vi "observacao_0MQ.vi"() -> ()   [LabVIEW 2012, in "Shared_160.lvlib"] (continued)
                        n2726 = call "Monta Comando.vi"("Set Point"=" 48 00", "Comando"="ESCREVER", "Dispositivo"="TAMPAS" ("Comando"), "Controlador"=w3460) -> ("Resposta"=w3454:string)  [unwired: 3 in, 2 out]
                        n2727 = Tick Count (ms)() -> (millisecond timer value=→"TF2":u32)
                        n2728 = Not Equal?(x=w3454, y="TAMPAS OK") -> ()  [unwired: 1 out]
                        n2729 = Select(t="REPOUSO" ("y"), s=FALSE, f="ESPERA2") -> (s? t:f=w3455:string)
                      }
                      frame "ESPERA2" {
                        # "10 SEGUNDOS"
                        n2730 = local read "TF2"() -> (w3461:u32)
                        n2731 = Tick Count (ms)() -> (millisecond timer value=w3467:u32)
                        n2732 = Add(x=w3461, y=u32 10000) -> (x+y=w3468:u32)
                        n2733 = Greater?(x=w3467, y=w3468) -> (0:w3462:bool)
                        n2734 = Select(t="PIZZA3" ("y"), s=w3462, f="ESPERA2" ("y")) -> (s? t:f=w3463:string)
                      }
                      frame "PIZZA3" {
                        w3479 = u16 3 items=["ZERO", "AH", "DEC", "TUBO", "CUP"] ("Controlador")
                        n2735 = call "Monta Comando.vi"("Set Point"=" 48 48", "Comando"="ESCREVER", "Dispositivo"="TAMPAS" ("Comando"), "Controlador"=w3479) -> ("Resposta"=w3474:string)  [unwired: 3 in, 2 out]
                        n2736 = case shown="True" "Case Constant\n(See Context Help) 12" {
                          frame False {
                          }
                          frame True {
                            n2737 = local write "LED ACTION"(FALSE ("LED ACTION")) -> ()
                          }
                        }
                        n2738 = Not Equal?(x=w3474, y="TAMPAS OK") -> ()  [unwired: 1 out]
                        n2739 = Select(t="REPOUSO" ("y"), s=FALSE, f="REPOUSO" ("y")) -> (s? t:f=w3471:string)
                      }
                      frame "REPOUSO" {
                      }
                    }
                    n2740 = local write "ESTADO FECHAR"(w3370) -> ()
                    n2741 = local read "ESTADO ABRIR"() -> (w3369:string)
                    n2742 = case shown="\"ESPERA3\"" w3369 {
                      tunnel: [w3376 w3384 w3392 w3402 w3411 w3424 "REPOUSO" ("y")] -> w3368
                      frame "INICIO", Default {
                        w3382 = u16 3 items=["ZERO", "AH", "DEC", "TUBO", "CUP"] ("Controlador")
                        # "PASSA PARA MODO HANDSET"
                        n2743 = call "Monta Comando.vi"("Set Point"=" F8 00", "Comando"="ESCREVER", "Dispositivo"="TAMPAS" ("Comando"), "Controlador"=w3382) -> ("Resposta"=w3377:string)  [unwired: 3 in, 2 out]
                        n2744 = Not Equal?(x=w3377, y="TAMPAS OK") -> ()  [unwired: 1 out]
                        n2745 = Tick Count (ms)() -> (millisecond timer value=→"TA1":u32)
                        n2746 = Select(t="REPOUSO" ("y"), s=FALSE, f="ESPERA1" ("y")) -> (s? t:f=w3376:string)
                      }
                      frame "ESPERA1" {
                        # "1 SEGUNDO"
                        n2747 = local read "TA1"() -> (w3383:u32)
                        n2748 = Tick Count (ms)() -> (millisecond timer value=w3389:u32)
                        n2749 = Add(x=w3383, y=u32 1000) -> (x+y=w3388:u32)
                        n2750 = Greater?(x=w3389, y=w3388) -> (0:w3386:bool)
                        n2751 = Select(t="ABREPIZZA" ("y"), s=w3386, f="ESPERA1" ("y")) -> (s? t:f=w3384:string)
                      }
                      frame "ABREPIZZA" {
                        w3401 = u16 3 items=["ZERO", "AH", "DEC", "TUBO", "CUP"] ("Controlador")
                        # "MANDA PIZZA ABRIR"
                        n2752 = call "Monta Comando.vi"("Set Point"=" 48 48", "Comando"="ESCREVER", "Dispositivo"="TAMPAS" ("Comando"), "Controlador"=w3401) -> ("Resposta"=w3396:string)  [unwired: 3 in, 2 out]
                        n2753 = Not Equal?(x=w3396, y="TAMPAS OK") -> ()  [unwired: 1 out]
                        n2754 = Tick Count (ms)() -> (millisecond timer value=→"TA2":u32)
                        n2755 = Select(t="ABREPIZZA" ("y"), s=FALSE, f="ESPERA2" ("y")) -> (s? t:f=w3392:string)
                      }
                      frame "ESPERA2" {
                        # "10 SEGUNDOS"
                        n2756 = local read "TA2"() -> (w3403:u32)
                        n2757 = Tick Count (ms)() -> (millisecond timer value=w3408:u32)
                        n2758 = Add(x=w3403, y=u32 10000) -> (x+y=w3407:u32)
                        n2759 = Greater?(x=w3408, y=w3407) -> (0:w3405:bool)
                        n2760 = Select(t="BACIAABRINDO" ("y"), s=w3405, f="ESPERA2" ("y")) -> (s? t:f=w3402:string)
                      }
                      frame "BACIAABRINDO" {
                        w3420 = u16 3 items=["ZERO", "AH", "DEC", "TUBO", "CUP"] ("Controlador")
                        # "BACIA ABRINDO"
                        n2761 = call "Monta Comando.vi"("Set Point"=" A0 20", "Comando"="ESCREVER", "Dispositivo"="TAMPAS" ("Comando"), "Controlador"=w3420) -> ("Resposta"=w3415:string)  [unwired: 3 in, 2 out]
                        n2762 = Not Equal?(x=w3415, y="TAMPAS OK") -> ()  [unwired: 1 out]
                        n2763 = Tick Count (ms)() -> (millisecond timer value=→"TA3":u32)
                        n2764 = Select(t="BACIAABRINDO" ("y"), s=FALSE, f="ESPERA3" ("y")) -> (s? t:f=w3411:string)
                      }
                      frame "ESPERA3" {
                        # "25 SEGUNDOS"
                        n2765 = local read "TA3"() -> (w3422:u32)
                        n2766 = Tick Count (ms)() -> (millisecond timer value=w3427:u32)
                        n2767 = Add(x=w3422, y=u32 25000) -> (x+y=w3426:u32)
                        n2768 = Greater?(x=w3427, y=w3426) -> (0:w3421:bool)
                        n2769 = case shown="True" w3421 {
                          frame False {
                          }
                          frame True {
                            n2770 = local write "LED ACTION"(TRUE ("LED ACTION")) -> ()
                          }
                        }
                        n2771 = Select(t="REPOUSO" ("y"), s=w3421, f="ESPERA3" ("y")) -> (s? t:f=w3424:string)
                      }
                      frame "REPOUSO" {
                      }
                    }
                    n2772 = local write "ESTADO ABRIR"(w3368) -> ()
                  }
                }
              }
              frame #2 {
                # "MÁQUINA DE ESTADOS PROTEÇÃO"
                n2773 = case shown="3" "M_PROT" {
                  selector: "M_PROT" -> [w3485 _ _ _ _ _]
                  tunnel: [w3485 w3486 w3505 5 5 ("estadoCUP") 0 ("estadoCUP")] -> w3483
                  frame 0, Default {
                    # "Sem movimento"
                    n2774 = call "TickTimeout.vi"() -> ("msTick"=→"Timeout PROT":u32)  [unwired: 2 in, 2 out]
                  }
                  frame 1 {
                    w3489 = u16 3 items=["Alarme", "Atencao", "Erro", "Ocupado", "Protecao", "Embreagem", "Tracking", "Var. Track", "Rápido", "Ligeiro", "Médio", "Lento", "Em movimento", ""] ("NomeStatus")
                    w3488 = u16 3 items=["Alarme", "Atencao", "Erro", "Ocupado", "Protecao", "Embreagem", "Tracking", "Var. Track", "Rápido", "Ligeiro", "Médio", "Lento", "Em movimento", ""] ("NomeStatus")
                    # "Testa Ocupado"
                    n2775 = call "Bit Status DEC.vi"("NomeStatus"=w3488) -> ("StatBit"=w3490:bool)
                    n2776 = call "Bit Status AH.vi"("NomeStatus"=w3489) -> ("StatBit"=w3491:bool)
                    n2777 = Or(x=w3491, y=w3490) -> (x .or. y?=w3487:bool)
                    n2778 = case shown="False" w3487 {
                      tunnel: [2 w3502] -> w3486
                      frame False {
                        w3498 = u16 2 items=["ZERO", "AH", "DEC", "TUBO", "CUP"] ("Controlador")
                        w3493 = u16 1 items=["ZERO", "AH", "DEC", "TUBO", "CUP"] ("Controlador")
                        # "Comando para os controladores\nsaírem da Proteção"
                        n2779 = call "Monta Comando.vi"("Comando"="LIBERAR", "Dispositivo"="EIXO" ("Comando"), "Controlador"=w3493) -> ()  [unwired: 4 in, 3 out]
                        n2780 = call "Monta Comando.vi"("Comando"="LIBERAR", "Dispositivo"="EIXO" ("Comando"), "Controlador"=w3498) -> ()  [unwired: 4 in, 3 out]
                      }
                      frame True {
                        # "Busy"
                        n2781 = local read "Timeout PROT"() -> (w3501:u32)
                        n2782 = call "TickTimeout.vi"("msInicial"=w3501, "msTimeout"=u32 20000) -> ("Timeout"=w3499:bool)  [unwired: 2 out]
                        n2783 = case shown="False" w3499 {
                          tunnel: [1 3] -> w3502
                          frame False {
                          }
                          frame True {
                          }
                        }
                      }
                    }
                  }
                  frame 2 {
                    # "Cálculos rápidos"
                    # "Vem do Setup"
                    # "Aguarda Sair da proteção"
                    n2784 = global read "Global_Telescopio.vi" "Zenital angle GRAUS"() -> (w3508:dbl)
                    n2785 = global read "Global_Telescopio.vi" "Z_LIBERA_GRAUS"() -> (w3507:dbl)
                    n2786 = Less?(x=w3508, y=w3507) -> (x < y?=w3506:bool)
                    n2787 = case shown="True" w3506 {
                      tunnel: [2 ("estadoCUP") 4 ("estadoCUP")] -> w3505
                      frame False {
                      }
                      frame True {
                        # "stop"
                      }
                    }
                  }
                  frame 3 {
                    w3511 = "TENTE NOVAMENTE" ("SYSTEM MESSAGES")
                    # "Trata Timeout"
                    n2788 = call "TickTimeout.vi"() -> ("msTick"=w3512:u32)  [unwired: 2 in, 2 out]
                    n2789 = call "Monta_Mensagem.vi"("Mensagem"=w3511) -> ()  [unwired: 2 in]
                    n2790 = call "Salva_systems_messages.vi"("Mensagem"=w3511) -> ()  [unwired: 5 in]
                    n2791 = local write "Timeout PROT"(w3512) -> ()
                  }
                  frame 4 {
                    w3515 = u16 1 items=["ZERO", "AH", "DEC", "TUBO", "CUP"] ("Controlador")
                    w3520 = u16 2 items=["ZERO", "AH", "DEC", "TUBO", "CUP"] ("Controlador")
                    # "Para os motores"
                    n2792 = call "Monta Comando.vi"("Comando"="PARAR", "Dispositivo"="PROG", "Controlador"=w3515) -> ()  [unwired: 4 in, 3 out]
                    n2793 = call "Monta Comando.vi"("Comando"="PARAR", "Dispositivo"="PROG", "Controlador"=w3520) -> ()  [unwired: 4 in, 3 out]
                  }
                  frame 5 {
                    # "SAÍDA"
                  }
                }
                n2794 = local write "M_PROT"(w3483) -> ()
              }
              frame #3 {
                w3539 = u16 3 items=["Alarme", "Atencao", "Erro", "Ocupado", "TBD", "LCB", "Trapeira", "Paravento", "DomoRap", "DomoCW", "DomoCCW", "TBD", "Em movimento", "TBD"] ("NomeStatus")
                w3545 = u16 3 items=["Alarme", "Atencao", "Erro", "Ocupado", "Protecao", "Embreagem", "Tracking", "Var. Track", "Rápido", "Ligeiro", "Médio", "Lento", "Em movimento", ""] ("NomeStatus")
                w3546 = u16 3 items=["Alarme", "Atencao", "Erro", "Ocupado", "Protecao", "Embreagem", "Tracking", "Var. Track", "Rápido", "Ligeiro", "Médio", "Lento", "Em movimento", ""] ("NomeStatus")
                n2795 = global read "Global_Telescopio.vi" "LimiarRapMed"() -> (w3547:dbl)
                n2796 = global read "Global_Telescopio.vi" "PosAH"() -> (w3549:dbl)
                n2797 = global read "Global_Telescopio.vi" "ErroMaxEixo"() -> (w3544:dbl)
                n2798 = global read "Global_Telescopio.vi" "PosDEC"() -> (w3548:dbl)
                n2799 = call "Bit Status DEC.vi"("NomeStatus"=w3545) -> ("StatBit"=w3543:bool)
                n2800 = call "Bit Status AH.vi"("NomeStatus"=w3546) -> ("StatBit"=w3542:bool)
                n2801 = case shown="4" "M_DEC" {
                  selector: "M_DEC" -> [w3642 _ _ _ _ _ _ _ _]
                  tunnel: [w3642 w3648 w3675 w3700 w3723 w3747 0 w3764 w3769] -> w3528
                  tunnel: "DestDEC" -> [_ w3647 w3672 w3694 w3720 _ _ _ _]
                  tunnel: w3548 -> [_ w3650 _ w3697 _ _ _ _ _]
                  tunnel: w3544 -> [_ _ _ w3698 _ _ _ _ _]
                  tunnel: w3547 -> [_ w3649 _ _ _ _ _ _ _]
                  tunnel: w3543 -> [_ w3646 _ w3693 _ _ _ _ _]
                  frame 0, Default {
                    w3640 = 0 ("CR DEC")
                    # "Sem apontamento"
                    n2802 = call "TickTimeout.vi"() -> ("msTick"=→"TimeoutDEC 2":u32)  [unwired: 2 in, 2 out]
                    "CR DEC UTILS" <- w3640
                    "CONT DEC UTILS" <- w3640
                  }
                  frame 1 {
                    # "Envia\nComando"
                    n2803 = Subtract(x=w3647, y=w3650) -> (x-y=w3645:dbl)
                    n2804 = Absolute Value(x=w3645) -> (abs(x)=w3651:dbl)
                    n2805 = Less?(x=w3651, y=w3649) -> (x < y?=w3644:bool)
                    n2806 = case shown="False" w3644 {
                      tunnel: [w3655 3] -> w3648
                      tunnel: w3647 -> [w3654 _]
                      tunnel: w3645 -> [w3653 _]
                      tunnel: w3646 -> [w3652 _]
                      frame False {
                        # "destino"
                        # "Fora do"
                        n2807 = case shown="False" w3652 {
                          tunnel: [20 w3664] -> w3655
                          tunnel: w3654 -> [w3658 _]
                          tunnel: w3653 -> [_ _]
                          frame False {
                            w3662 = u16 2 items=["ZERO", "AH", "DEC", "TUBO", "CUP"] ("Controlador")
                            # "CLP Pronto"
                            n2808 = local write "DEC on Target"(FALSE ("DEC on Target")) -> ()
                            n2809 = call "rad_hms.vi"("TRUE=HORA\nFALSE=GRAU"=FALSE, "Radiano"=w3658) -> ("Hora/Graus Texto Decimal"=w3659:string)  [unwired: 3 in]
                            n2810 = call "Monta Comando.vi"("Set Point"=w3659, "Comando"="MOVER_RAP", "Dispositivo"="EIXO" ("Comando"), "Controlador"=w3662) -> ()  [unwired: 3 in, 3 out]
                          }
                          frame True {
                            # "CLP Ocupado"
                            n2811 = local read "TimeoutDEC 2"() -> (w3666:u32)
                            n2812 = call "TickTimeout.vi"("msInicial"=w3666, "msTimeout"=u32 4000) -> ("Timeout"=w3665:bool)  [unwired: 2 out]
                            n2813 = case shown="False" w3665 {
                              tunnel: [1 5] -> w3664
                              frame False {
                              }
                              frame True {
                                # "Tratar\nTimeout"
                              }
                            }
                          }
                        }
                      }
                      frame True {
                        # "Dist. pequena p/ mov. rápido"
                        # "Ligar mov. lento"
                        n2814 = call "TickTimeout.vi"() -> ("msTick"=w3670:u32)  [unwired: 2 in, 2 out]
                        n2815 = local write "TimeoutDEC 2"(w3670) -> ()
                      }
                    }
                    n2816 = local write "dec="(FALSE ("dec=")) -> ()
                  }
                  frame 2 {
                    w3678 = u16 12 items=["Alarme", "Atencao", "Erro", "Ocupado", "Protecao", "Embreagem", "Tracking", "Var. Track", "Rápido", "Ligeiro", "Médio", "Lento", "Em movimento", ""] ("NomeStatus")
                    # "Aguarda fim mov. Rap."
                    n2817 = call "Bit Status DEC.vi"("NomeStatus"=w3678) -> ("StatBit"=w3679:bool)
                    n2818 = case shown="False" w3679 {
                      tunnel: [1 w3688] -> w3676
                      tunnel: w3672 -> [_ w3687]
                      frame False {
                        # "Motor parado.\nTestar se chegou\nao destino"
                        n2819 = call "TickTimeout.vi"() -> ("msTick"=w3684:u32)  [unwired: 2 in, 2 out]
                        n2820 = local write "TimeoutDEC 2"(w3684) -> ()
                      }
                      frame True {
                        # "Ainda movendo...\nAGUARDAR"
                        n2821 = call "PROTECAO_DEC_UTILS.vi"("Destino DEC"=w3687) -> ("CONT DEC"=w3686:i32)  [unwired: 10 in]
                        n2822 = local read "Erro PROTEC"() -> (w3689:i32)
                        n2823 = Greater Or Equal?(x=w3686, y=w3689) -> (x >= y?=w3692:bool)
                        n2824 = local write "CONT DEC UTILS"(w3686) -> ()
                        n2825 = Select(t=6, s=w3692, f=2) -> (s? t:f=w3688:i32)
                      }
                    }
                    n2826 = global read "Global_Telescopio.vi" "Habilita supervisao"() -> (w3674:bool)
                    n2827 = case shown="True" w3674 {
                      tunnel: [FALSE w3683] -> w3673
                      frame False {
                      }
                      frame True {
                        n2828 = local read "CR DEC UTILS"() -> (w3681:i32)
                        n2829 = local read "Erro Lim"() -> (w3682:i32)
                        n2830 = Greater Or Equal?(x=w3681, y=w3682) -> (x >= y?=w3683:bool)
                      }
                    }
                    n2831 = Select(t=6, s=w3673, f=w3676) -> (s? t:f=w3675:i32)
                  }
                  frame 3 {
                    # "Mov.Lento"
                    n2832 = Subtract(x=w3694, y=w3697) -> (x-y=w3695:dbl)
                    n2833 = Absolute Value(x=w3695) -> (abs(x)=w3699:dbl)
                    n2834 = Less Or Equal?(x=w3699, y=w3698) -> (x <= y?=w3696:bool)
                    n2835 = case shown="False" w3696 {
                      tunnel: [w3702 0] -> w3700
                      tunnel: w3695 -> [w3701 _]
                      tunnel: w3693 -> [w3703 _]
                      frame False {
                        n2836 = case shown="False" w3703 {
                          tunnel: [40 w3712] -> w3702
                          tunnel: w3701 -> [w3706 _]
                          frame False {
                            w3711 = u16 2 items=["ZERO", "AH", "DEC", "TUBO", "CUP"] ("Controlador")
                            # "Mov. lento"
                            n2837 = call "TickTimeout.vi"() -> ("msTick"=w3704:u32)  [unwired: 2 in, 2 out]
                            n2838 = local write "TimeoutDEC 2"(w3704) -> ()
                            n2839 = call "rad_hms.vi"("TRUE=HORA\nFALSE=GRAU"=FALSE ("TRUE=HORA\nFALSE=GRAU"), "Radiano"=w3706) -> ("Hora/Graus Texto Decimal"=w3708:string)  [unwired: 3 in]
                            n2840 = call "Monta Comando.vi"("Set Point"=w3708, "Comando"="MOVER_REL", "Dispositivo"="EIXO" ("Comando"), "Controlador"=w3711) -> ()  [unwired: 3 in, 3 out]
                          }
                          frame True {
                            # "CLP Ocupado"
                            n2841 = local read "TimeoutDEC 2"() -> (w3714:u32)
                            n2842 = call "TickTimeout.vi"("msInicial"=w3714, "msTimeout"=u32 2000) -> ("Timeout"=w3713:bool)  [unwired: 2 out]
                            n2843 = case shown="False" w3713 {
                              tunnel: [3 5] -> w3712
                              frame False {
                              }
                              frame True {
                              }
                            }
                          }
                        }
                      }
                      frame True {
                        # "DEC no destino"
                        n2844 = local write "DEC on Target"(TRUE ("DEC on Target")) -> ()
                      }
                    }
                  }
                  frame 4 {
                    w3726 = u16 12 items=["Alarme", "Atencao", "Erro", "Ocupado", "Protecao", "Embreagem", "Tracking", "Var. Track", "Rápido", "Ligeiro", "Médio", "Lento", "Em movimento", ""] ("NomeStatus")
                    # "Aguarda fim mov. lento"
                    n2845 = global read "Global_Telescopio.vi" "Habilita supervisao"() -> (w3725:bool)
                    n2846 = call "Bit Status DEC.vi"("NomeStatus"=w3726) -> ("StatBit"=w3727:bool)
                    n2847 = case shown="True" w3727 {
                      tunnel: [3 w3737] -> w3722
                      tunnel: w3720 -> [_ w3735]
                      frame False {
                        # "Motor parado.\nTestar se chegou\nao destino"
                        n2848 = call "TickTimeout.vi"() -> ("msTick"=w3732:u32)  [unwired: 2 in, 2 out]
                        n2849 = local write "TimeoutDEC 2"(w3732) -> ()
                      }
                      frame True {
                        n2850 = call "PROTECAO_DEC_UTILS.vi"("Destino DEC"=w3735) -> ("CONT DEC"=w3734:i32)  [unwired: 10 in]
                        n2851 = local read "Erro PROTEC"() -> (w3740:i32)
                        n2852 = local write "CONT DEC UTILS"(w3734) -> ()
                        n2853 = Greater Or Equal?(x=w3734, y=w3740) -> (x >= y?=w3742:bool)
                        n2854 = local read "TimeoutDEC 2"() -> (w3736:u32)
                        n2855 = call "TickTimeout.vi"("msInicial"=w3736, "msTimeout"=u32 4000) -> ("Timeout"=w3739:bool)  [unwired: 2 out]
                        n2856 = case shown="False" w3739 {
                          tunnel: [4 5] -> w3743
                          frame False {
                          }
                          frame True {
                          }
                        }
                        n2857 = Select(t=6, s=w3742, f=w3743) -> (s? t:f=w3737:i32)
                      }
                    }
                    n2858 = case shown="True" w3725 {
                      tunnel: [FALSE w3731] -> w3721
                      frame False {
                      }
                      frame True {
                        n2859 = local read "CR DEC UTILS"() -> (w3729:i32)
                        n2860 = local read "Erro Lim"() -> (w3730:i32)
                        n2861 = Greater Or Equal?(x=w3729, y=w3730) -> (x >= y?=w3731:bool)
                      }
                    }
                    n2862 = Select(t=6, s=w3721, f=w3722) -> (s? t:f=w3723:i32)
                  }
                  frame 5 {
                    w3753 = u16 2 items=["ZERO", "AH", "DEC", "TUBO", "CUP"] ("Controlador")
                    # "Reiniciar apontamento"
                    # "Trata Timeout"
                    n2863 = call "TickTimeout.vi"() -> ("msTick"=w3746:u32)  [unwired: 2 in, 2 out]
                    n2864 = local write "TimeoutDEC 2"(w3746) -> ()
                    n2865 = call "Monta Comando.vi"("Comando"="PARAR", "Dispositivo"="PROG" ("Comando"), "Controlador"=w3753) -> ("Erro Comunicação"=w3748:bool)  [unwired: 4 in, 2 out]
                    n2866 = Select(t=6, s=w3748, f=1) -> (s? t:f=w3747:i32)
                  }
                  frame 6 {
                    n2867 = stacked-sequence {
                      frame #0 {
                        w3758 = u16 2 items=["ZERO", "AH", "DEC", "TUBO", "CUP"] ("Controlador")
                        # "Trata Timeout"
                        n2868 = local write "dec="(TRUE ("dec=")) -> ()
                        n2869 = call "Monta Comando.vi"("Comando"="PARAR", "Dispositivo"="PROG" ("Comando"), "Controlador"=w3758) -> ()  [unwired: 4 in, 3 out]
                      }
                      frame #1 {
                        w3760 = "Erro de Controlador DEC , REAPONTAR !" ("Mensagem")
                        n2870 = local write "Flag de erro p/ apagar lampada"(TRUE ("Flag de erro p/ apagar lampada")) -> ()
                        n2871 = call "Monta_Mensagem.vi"("Mensagem"=w3760) -> ()  [unwired: 2 in]
                        n2872 = call "Salva_systems_messages.vi"("Mensagem"=w3760) -> ()  [unwired: 5 in]
                      }
                      frame #2 {
                        w3762 = u16 2 items=["ZERO", "AH", "DEC", "TUBO", "CUP"] ("Controlador")
                        # "Em movimento não aceita reset"
                        # "Segundo PARAR por garantia"
                        n2873 = call "Monta Comando.vi"("Comando"="PARAR", "Dispositivo"="PROG", "Controlador"=w3762) -> ()  [unwired: 4 in, 3 out]
                      }
                    }
                  }
                  frame 20 {
                    # "Espera entrar\nem movimento"
                    n2874 = local read "Flag ativo DEC"() -> (w3765:bool)
                    n2875 = case shown="True" w3765 {
                      tunnel: [20 ("t") 2 ("t")] -> w3764
                      frame False {
                      }
                      frame True {
                        # "limpa flag"
                        n2876 = local write "Flag ativo DEC"(FALSE ("Flag ativo AH")) -> ()
                      }
                    }
                  }
                  frame 40 {
                    # "Espera entrar\nem movimento"
                    n2877 = local read "Flag ativo DEC"() -> (w3770:bool)
                    n2878 = case shown="True" w3770 {
                      tunnel: [40 ("t") 4 ("t")] -> w3769
                      frame False {
                      }
                      frame True {
                        # "limpa flag"
                        n2879 = local write "Flag ativo DEC"(FALSE ("Flag ativo AH")) -> ()
                      }
                    }
                  }
                }
                n2880 = case shown="6" "M_AH" {
                  selector: "M_AH" -> [w3776 _ _ _ _ _ _ _ _ _ _]
                  tunnel: [w3776 w3777 w3797 w3828 5 w3851 w3880 w3902 0 w3920 w3925] -> w3530
                  tunnel: "DestAH" -> [_ _ w3794 w3824 _ w3847 w3876 _ _ _ _]
                  tunnel: w3549 -> [_ _ w3800 _ _ w3853 _ _ _ _ _]
                  tunnel: w3544 -> [_ _ _ _ _ w3852 _ _ _ _ _]
                  tunnel: w3547 -> [_ _ w3801 _ _ _ _ _ _ _ _]
                  tunnel: w3542 -> [_ w3778 w3795 _ _ w3849 _ _ _ _ _]
                  frame 0, Default {
                    w3774 = 0 ("CR AH")
                    # "Sem apontamento"
                    n2881 = call "TickTimeout.vi"() -> ("msTick"=→"TimeoutAH 2":u32)  [unwired: 2 in, 2 out]
                    "CR AH UTILS" <- w3774
                    "CONT AH UTILS" <- w3774
                  }
                  frame 1 {
                    n2882 = case shown="False" w3778 {
                      tunnel: [2 w3788] -> w3777
                      frame False {
                        n2883 = stacked-sequence {
                          frame #0 {
                            w3783 = u16 1 items=["ZERO", "AH", "DEC", "TUBO", "CUP"] ("Controlador")
                            # "Desliga Acomp Sideral"
                            n2884 = call "Monta Comando.vi"("Comando"="DESLIGAR", "Dispositivo"="SIDERAL" ("Comando"), "Controlador"=w3783) -> ()  [unwired: 4 in, 3 out]
                          }
                          frame #1 {
                            w3786 = u16 1 items=["ZERO", "AH", "DEC", "TUBO", "CUP"] ("Controlador")
                            # "Parar Eixo AH"
                            n2885 = call "Monta Comando.vi"("Comando"="PARAR", "Dispositivo"="PROG" ("Comando"), "Controlador"=w3786) -> ()  [unwired: 4 in, 3 out]
                          }
                        }
                        n2886 = call "TickTimeout.vi"() -> ("msTick"=w3779:u32)  [unwired: 2 in, 2 out]
                        n2887 = local write "TimeoutAH 2"(w3779) -> ()
                      }
                      frame True {
                        n2888 = local read "TimeoutAH 2"() -> (w3787:u32)
                        n2889 = call "TickTimeout.vi"("msInicial"=w3787, "msTimeout"=u32 5000) -> ("Timeout"=w3790:bool)  [unwired: 2 out]
                        n2890 = case shown="False" w3790 {
                          tunnel: [1 7] -> w3788
                          frame False {
                          }
                          frame True {
                          }
                        }
                      }
                    }
                  }
                  frame 2 {
                    # "Mov.Rapido"
                    n2891 = Subtract(x=w3794, y=w3800) -> (x-y=w3798:dbl)
                    n2892 = Absolute Value(x=w3798) -> (abs(x)=w3799:dbl)
                    n2893 = Less?(x=w3799, y=w3801) -> (x < y?=w3796:bool)
                    n2894 = case shown="False" w3796 {
                      tunnel: w3794 -> [w3802 _]
                      tunnel: w3798 -> [_ _]
                      tunnel: [w3803 4] -> w3797
                      tunnel: w3795 -> [w3804 _]
                      frame False {
                        n2895 = case shown="False" w3804 {
                          tunnel: w3802 -> [w3810 _]
                          tunnel: [w3805 w3816] -> w3803
                          frame False {
                            w3812 = u16 1 items=["ZERO", "AH", "DEC", "TUBO", "CUP"] ("Controlador")
                            # "Aguardar\nfim mov."
                            # "Mov. rápido"
                            n2896 = local write "RA on Target"(FALSE ("RA on Target")) -> ()
                            n2897 = call "rad_hms.vi"("TRUE=HORA\nFALSE=GRAU"=TRUE ("TRUE=HORA\nFALSE=GRAU"), "Radiano"=w3810) -> ("Hora/Graus Texto Decimal"=w3815:string)  [unwired: 3 in]
                            n2898 = call "Monta Comando.vi"("Set Point"=w3815, "Comando"="MOVER_RAP", "Dispositivo"="EIXO" ("Comando"), "Controlador"=w3812) -> ("Erro Comunicação"=w3806:bool)  [unwired: 3 in, 2 out]
                            n2899 = Select(t=8, s=w3806, f=30) -> (s? t:f=w3805:i32)
                          }
                          frame True {
                            # "CLP Ocupado"
                            n2900 = local read "TimeoutAH 2"() -> (w3818:u32)
                            n2901 = call "TickTimeout.vi"("msInicial"=w3818, "msTimeout"=u32 4000) -> ("Timeout"=w3817:bool)  [unwired: 2 out]
                            n2902 = case shown="True" w3817 {
                              tunnel: [2 7] -> w3816
                              frame False {
                              }
                              frame True {
                                # "Tratar\nTimeout"
                              }
                            }
                          }
                        }
                      }
                      frame True {
                        # "Dist. pequena p/ mov. rápido"
                        n2903 = call "TickTimeout.vi"() -> ("msTick"=w3822:u32)  [unwired: 2 in, 2 out]
                        n2904 = local write "TimeoutAH 2"(w3822) -> ()
                      }
                    }
                    n2905 = local write "ah="(FALSE ("ah=")) -> ()
                  }
                  frame 3 {
                    w3831 = u16 12 items=["Alarme", "Atencao", "Erro", "Ocupado", "Protecao", "Embreagem", "Tracking", "Var. Track", "Rápido", "Ligeiro", "Médio", "Lento", "Em movimento", ""] ("NomeStatus")
                    # "Aguarda fim mov. Rap."
                    n2906 = call "Bit Status AH.vi"("NomeStatus"=w3831) -> ("StatBit"=w3830:bool)
                    n2907 = case shown="True" w3830 {
                      tunnel: [2 w3840] -> w3827
                      tunnel: w3824 -> [_ w3839]
                      frame False {
                        # "Motor parado.\nTestar se precisa\nde novo cmd. \nde mov. rápido"
                        n2908 = call "TickTimeout.vi"() -> ("msTick"=w3836:u32)  [unwired: 2 in, 2 out]
                        n2909 = local write "TimeoutAH 2"(w3836) -> ()
                      }
                      frame True {
                        # "Aqui também \ncaberia um \nTimeout?"
                        # "Ainda movendo...\nAGUARDAR"
                        n2910 = call "PROTECAO_AH_UTILS.vi"("DestinoAH"=w3839) -> ("CONT AH"=w3838:i32)  [unwired: 10 in]
                        n2911 = local read "Erro PROTEC"() -> (w3842:i32)
                        n2912 = local write "CONT AH UTILS"(w3838) -> ()
                        n2913 = Greater Or Equal?(x=w3838, y=w3842) -> (x >= y?=w3843:bool)
                        n2914 = Select(t=8, s=w3843, f=3) -> (s? t:f=w3840:i32)
                      }
                    }
                    n2915 = global read "Global_Telescopio.vi" "Habilita supervisao"() -> (w3826:bool)
                    n2916 = case shown="True" w3826 {
                      tunnel: [FALSE w3835] -> w3825
                      frame False {
                      }
                      frame True {
                        n2917 = local read "Erro Lim"() -> (w3834:i32)
                        n2918 = local read "CR AH UTILS"() -> (w3833:i32)
                        n2919 = Greater Or Equal?(x=w3833, y=w3834) -> (x >= y?=w3835:bool)
                      }
                    }
                    n2920 = Select(t=8, s=w3825, f=w3827) -> (s? t:f=w3828:i32)
                  }
                  frame 4 {
                    # "Não faz nada"
                    n2921 = call "TickTimeout.vi"() -> ("msTick"=w3846:u32)  [unwired: 2 in, 2 out]
                    n2922 = local write "TimeoutAH 2"(w3846) -> ()
                  }
                  frame 5 {
                    # "Mov.Lento"
                    n2923 = Subtract(x=w3847, y=w3853) -> (x-y=w3848:dbl)
                    n2924 = Absolute Value(x=w3848) -> (abs(x)=w3854:dbl)
                    n2925 = Less Or Equal?(x=w3854, y=w3852) -> (x <= y?=w3850:bool)
                    n2926 = case shown="True" w3850 {
                      tunnel: w3848 -> [w3856 _]
                      tunnel: [w3855 0] -> w3851
                      tunnel: w3849 -> [w3857 _]
                      frame False {
                        n2927 = case shown="False" w3857 {
                          tunnel: w3856 -> [w3862 _]
                          tunnel: [w3861 w3868] -> w3855
                          frame False {
                            w3864 = u16 1 items=["ZERO", "AH", "DEC", "TUBO", "CUP"] ("Controlador")
                            # "Envia Cmd. Mov. Lento"
                            n2928 = call "rad_hms.vi"("TRUE=HORA\nFALSE=GRAU"=TRUE ("TRUE=HORA\nFALSE=GRAU"), "Radiano"=w3862) -> ("Hora/Graus Texto Decimal"=w3867:string)  [unwired: 3 in]
                            n2929 = call "Monta Comando.vi"("Set Point"=w3867, "Comando"="MOVER_REL", "Dispositivo"="EIXO" ("Comando"), "Controlador"=w3864) -> ("Erro Comunicação"=w3859:bool)  [unwired: 3 in, 2 out]
                            n2930 = Select(t=8, s=w3859, f=60) -> (s? t:f=w3861:i32)
                          }
                          frame True {
                            # "CLP Ocupado"
                            n2931 = local read "TimeoutAH 2"() -> (w3870:u32)
                            n2932 = call "TickTimeout.vi"("msInicial"=w3870, "msTimeout"=u32 4000) -> ("Timeout"=w3869:bool)  [unwired: 2 out]
                            n2933 = case shown="False" w3869 {
                              tunnel: [5 7] -> w3868
                              frame False {
                              }
                              frame True {
                              }
                            }
                          }
                        }
                      }
                      frame True {
                        # "AH on Target"
                        n2934 = local write "RA on Target"(TRUE ("RA on Target")) -> ()
                      }
                    }
                  }
                  frame 6 {
                    w3883 = u16 12 items=["Alarme", "Atencao", "Erro", "Ocupado", "Protecao", "Embreagem", "Tracking", "Var. Track", "Rápido", "Ligeiro", "Médio", "Lento", "Em movimento", ""] ("NomeStatus")
                    # "Aguarda fim mov. Lento"
                    n2935 = call "Bit Status AH.vi"("NomeStatus"=w3883) -> ("StatBit"=w3882:bool)
                    n2936 = case shown="True" w3882 {
                      tunnel: [5 w3897] -> w3879
                      tunnel: w3876 -> [_ w3891]
                      frame False {
                        # "Motor parado.\nTestar se chegou\nao destino"
                        n2937 = call "TickTimeout.vi"() -> ("msTick"=w3888:u32)  [unwired: 2 in, 2 out]
                        n2938 = local write "TimeoutAH 2"(w3888) -> ()
                      }
                      frame True {
                        n2939 = local read "Erro PROTEC"() -> (w3899:i32)
                        n2940 = call "PROTECAO_AH_UTILS.vi"("DestinoAH"=w3891) -> ("CONT AH"=w3890:i32)  [unwired: 10 in]
                        n2941 = local write "CONT AH UTILS"(w3890) -> ()
                        n2942 = local read "TimeoutAH 2"() -> (w3892:u32)
                        n2943 = Greater Or Equal?(x=w3890, y=w3899) -> (x >= y?=w3893:bool)
                        n2944 = call "TickTimeout.vi"("msInicial"=w3892, "msTimeout"=u32 4000) -> ("Timeout"=w3896:bool)  [unwired: 2 out]
                        n2945 = case shown="False" w3896 {
                          tunnel: [6 7] -> w3894
                          frame False {
                          }
                          frame True {
                            # "Tratar\nTimeout"
                          }
                        }
                        n2946 = Select(t=8, s=w3893, f=w3894) -> (s? t:f=w3897:i32)
                      }
                    }
                    n2947 = global read "Global_Telescopio.vi" "Habilita supervisao"() -> (w3878:bool)
                    n2948 = case shown="True" w3878 {
                      tunnel: [FALSE w3887] -> w3877
                      frame False {
                      }
                      frame True {
                        n2949 = local read "CR AH UTILS"() -> (w3885:i32)
                        n2950 = local read "Erro Lim"() -> (w3886:i32)
                        n2951 = Greater Or Equal?(x=w3885, y=w3886) -> (x >= y?=w3887:bool)
                      }
                    }
                    n2952 = Select(t=8, s=w3877, f=w3879) -> (s? t:f=w3880:i32)
                  }
                  frame 7 {
                    w3907 = u16 1 items=["ZERO", "AH", "DEC", "TUBO", "CUP"] ("Controlador")
                    # "Reiniciar apontamento"
                    # "Trata Timeout"
                    n2953 = call "TickTimeout.vi"() -> ("msTick"=w3906:u32)  [unwired: 2 in, 2 out]
                    n2954 = local write "TimeoutAH 2"(w3906) -> ()
                    n2955 = call "Monta Comando.vi"("Comando"="PARAR", "Dispositivo"="PROG" ("Comando"), "Controlador"=w3907) -> ("Erro Comunicação"=w3903:bool)  [unwired: 4 in, 2 out]
                    n2956 = Select(t=8, s=w3903, f=2) -> (s? t:f=w3902:i32)
                  }
                  frame 8 {
                    n2957 = stacked-sequence {
                      frame #0 {
                        w3912 = u16 1 items=["ZERO", "AH", "DEC", "TUBO", "CUP"] ("Controlador")
                        # "Reiniciar apontamento"
                        # "Trata Timeout"
                        n2958 = local write "ah="(TRUE ("ah=")) -> ()
                        n2959 = call "Monta Comando.vi"("Comando"="PARAR", "Dispositivo"="PROG" ("Comando"), "Controlador"=w3912) -> ()  [unwired: 4 in, 3 out]
                      }
                      frame #1 {
                        w3916 = "Erro de Controlador RA , REAPONTAR !" ("Mensagem")
                        n2960 = local write "Flag de erro p/ apagar lampada"(TRUE ("Flag de erro p/ apagar lampada")) -> ()
                        n2961 = call "Monta_Mensagem.vi"("Mensagem"=w3916) -> ()  [unwired: 2 in]
                        n2962 = call "Salva_systems_messages.vi"("Mensagem"=w3916) -> ()  [unwired: 5 in]
                      }
                      frame #2 {
                        w3919 = u16 1 items=["ZERO", "AH", "DEC", "TUBO", "CUP"] ("Controlador")
                        # "Em movimento não aceita reset"
                        # "Segundo PARAR por garantia"
                        n2963 = call "Monta Comando.vi"("Comando"="PARAR", "Dispositivo"="PROG", "Controlador"=w3919) -> ()  [unwired: 4 in, 3 out]
                      }
                    }
                  }
                  frame 30 {
                    # "Espera entrar\nem movimento"
                    n2964 = local read "Flag ativo AH"() -> (w3921:bool)
                    n2965 = case shown="True" w3921 {
                      tunnel: [30 ("t") 3 ("t")] -> w3920
                      frame False {
                      }
                      frame True {
                        # "limpa flag"
                        n2966 = local write "Flag ativo AH"(FALSE ("Flag ativo AH")) -> ()
                      }
                    }
                  }
                  frame 60 {
                    # "Espera entrar\nem movimento"
                    n2967 = local read "Flag ativo AH"() -> (w3926:bool)
                    n2968 = case shown="True" w3926 {
                      tunnel: [60 ("t") 6 ("t")] -> w3925
                      frame False {
                      }
                      frame True {
                        # "limpa flag"
                        n2969 = local write "Flag ativo AH"(FALSE ("Flag ativo AH")) -> ()
                      }
                    }
                  }
                }
                n2970 = call "PROTECAO.vi"("Estado In"=w3530) -> ("Estado Out"=w3529:i32)  [unwired: 2 in]
                n2971 = call "PROTECAO.vi"("Estado In"=w3528) -> ("Estado Out"=w3527:i32)  [unwired: 2 in]
                n2972 = local read "M_PROT"() -> (w3524:i32)
                n2973 = property on="Setup, Pointing & Guiding" class="TabCtl (strict)"() -> ("Page Selector Visible"=w3534:bool)  [unwired: 2 in, 2 out]
                n2974 = call "Bit Status CUP.vi"("NomeStatus"=w3539) -> ("StatBit"=w3541:bool)
                n2975 = local write "M_DEC"(w3527) -> ()
                n2976 = Not(x=w3534) -> (.not. x?=w3532:bool)
                n2977 = case shown="2" "M_CUP" {
                  selector: "M_CUP" -> [w3554 _ _ _ _ _ _ _ _]
                  tunnel: [w3554 w3559 w3586 1 w3597 w3611 w3616 w3633 0 ("estadoCUP")] -> w3526
                  tunnel: w3541 -> [_ w3560 _ _ w3596 _ w3617 _ _]
                  tunnel: "DestCUP" -> [_ w3558 _ _ _ _ _ _ _]
                  frame 0, Default {
                    # "Sem movimento"
                    n2978 = call "TickTimeout.vi"() -> ("msTick"=→"TimeoutCUP 2":u32)  [unwired: 2 in, 2 out]
                  }
                  frame 1 {
                    # "20240820"
                    # "Envia\nComando"
                    n2979 = call "Checa destino cupula.vi"("Target"=w3558) -> ("moverCup"=w3557:bool, "angTarget"=w3555:string)  [unwired: 6 in, 1 out]
                    n2980 = Not(x=w3557) -> (.not. x?=w3556:bool)
                    n2981 = case shown="False" w3556 {
                      tunnel: w3560 -> [w3564 _]
                      tunnel: w3558 -> [w3563 _]
                      tunnel: [w3562 w3580] -> w3559
                      tunnel: w3555 -> [w3561 _]
                      frame False {
                        # "CUP fora pos."
                        n2982 = case shown="False" w3564 {
                          tunnel: w3563 -> [w3573 _]
                          tunnel: [2 w3574] -> w3562
                          tunnel: w3561 -> [w3565 _]
                          frame False {
                            w3570 = u16 4 items=["ZERO", "AH", "DEC", "TUBO", "CUP"] ("Controlador")
                            # "CLP Pronto"
                            n2983 = call "TickTimeout.vi"() -> ("msTick"=w3569:u32)  [unwired: 2 in, 2 out]
                            n2984 = Number To Decimal String(number=w3573) -> (decimal integer string=w3566:string)  [unwired: 1 in]
                            n2985 = local write "TimeoutCUP 2"(w3569) -> ()
                            n2986 = local write "Dome on Target"(FALSE ("Dome on Target")) -> ()
                            n2987 = local write "TargetCup"(w3565) -> ()
                            n2988 = call "Monta Comando.vi"("Set Point"=w3566, "Comando"="MOVER", "Dispositivo"="DOMO" ("Comando"), "Controlador"=w3570) -> ()  [unwired: 3 in, 3 out]
                          }
                          frame True {
                            # "CLP Busy"
                            n2989 = local read "TimeoutCUP 2"() -> (w3576:u32)
                            n2990 = call "TickTimeout.vi"("msInicial"=w3576, "msTimeout"=u32 5000) -> ("Timeout"=w3575:bool)  [unwired: 2 out]
                            n2991 = case shown="True" w3575 {
                              tunnel: [1 3] -> w3574
                              frame False {
                              }
                              frame True {
                              }
                            }
                          }
                        }
                      }
                      frame True {
                        # "Verifica\nTrapeira e\nParavento"
                        # "CUP no destino"
                        n2992 = call "TickTimeout.vi"() -> ("msTick"=w3584:u32)  [unwired: 2 in, 2 out]
                        n2993 = global read "Global_Telescopio.vi" "Parking"() -> (w3583:bool)
                        n2994 = local write "TimeoutCUP 2"(w3584) -> ()
                        n2995 = Select(t=4, s=w3583, f=8) -> (s? t:f=w3580:i32)
                      }
                    }
                  }
                  frame 2 {
                    w3585 = u16 12 items=["Alarme", "Atencao", "Erro", "Ocupado", "TBD", "LCB", "Trapeira", "Paravento", "DomoRap", "DomoCW", "DomoCCW", "TBD", "Em movimento", "TBD"] ("NomeStatus")
                    # "Aqui também caberia um Timeout?"
                    # "Aguarda parada motor"
                    n2996 = call "Bit Status CUP.vi"("NomeStatus"=w3585) -> ("StatBit"=w3587:bool)
                    n2997 = case shown="True" w3587 {
                      tunnel: [1 2] -> w3586
                      frame False {
                        # "Motor parado.\nTestar se chegou\nao destino"
                        n2998 = call "TickTimeout.vi"() -> ("msTick"=w3588:u32)  [unwired: 2 in, 2 out]
                        n2999 = local write "TimeoutCUP 2"(w3588) -> ()
                      }
                      frame True {
                        # "Ainda movendo...\nAGUARDAR"
                      }
                    }
                  }
                  frame 3 {
                    w3594 = u16 4 items=["ZERO", "AH", "DEC", "TUBO", "CUP"] ("Controlador")
                    # "Trata Timeout"
                    n3000 = call "TickTimeout.vi"() -> ("msTick"=w3591:u32)  [unwired: 2 in, 2 out]
                    n3001 = local write "TimeoutCUP 2"(w3591) -> ()
                    n3002 = call "Monta Comando.vi"("Comando"="PARAR", "Dispositivo"="PROG" ("Comando"), "Controlador"=w3594) -> ()  [unwired: 4 in, 3 out]
                  }
                  frame 4 {
                    # "Verifica Trapeira"
                    n3003 = case shown="True" w3596 {
                      tunnel: [5 w3602] -> w3597
                      frame False {
                        w3601 = u16 4 items=["ZERO", "AH", "DEC", "TUBO", "CUP"] ("Controlador")
                        # "Fechar Trapeira"
                        # "Aguardar abertura Trap."
                        # "CLP Pronto"
                        n3004 = call "Monta Comando.vi"("Comando"="FECHAR", "Dispositivo"="TRAPEIRA" ("Comando"), "Controlador"=w3601) -> ()  [unwired: 4 in, 3 out]
                      }
                      frame True {
                        # "CLP Busy"
                        n3005 = local read "TimeoutCUP 2"() -> (w3604:u32)
                        n3006 = call "TickTimeout.vi"("msInicial"=w3604, "msTimeout"=u32 5000) -> ("Timeout"=w3603:bool)  [unwired: 2 out]
                        n3007 = case shown="False" w3603 {
                          tunnel: [4 3] -> w3602
                          frame False {
                          }
                          frame True {
                          }
                        }
                      }
                    }
                  }
                  frame 5 {
                    w3609 = u16 6 items=["Alarme", "Atencao", "Erro", "Ocupado", "TBD", "LCB", "Trapeira", "Paravento", "DomoRap", "DomoCW", "DomoCCW", "TBD", "Em movimento", "TBD"] ("NomeStatus")
                    # "Aqui também caberia um Timeout?"
                    # "Aguarda Fechamento da Trapeira"
                    # "Também poderia ser testado o bit \"Em movimento\".\nNeste caso o código do \"IF\" deve ser permutado."
                    n3008 = call "Bit Status CUP.vi"("NomeStatus"=w3609) -> ("StatBit"=w3610:bool)
                    n3009 = Not(x=w3610) -> (.not. x?=w3608:bool)
                    n3010 = case shown="False" w3608 {
                      tunnel: [5 6] -> w3611
                      frame False {
                        # "Ainda movendo...\nAGUARDAR"
                      }
                      frame True {
                        # "Trapeira Fechada.\nVerificar Paravento."
                        n3011 = call "TickTimeout.vi"() -> ("msTick"=w3613:u32)  [unwired: 2 in, 2 out]
                        n3012 = local write "TimeoutCUP 2"(w3613) -> ()
                      }
                    }
                  }
                  frame 6 {
                    # "Verifica Paravento"
                    n3013 = case shown="True" "Case Ct" {
                      tunnel: w3617 -> [_ w3620]
                      tunnel: [8 w3619] -> w3616
                      frame False {
                        # "Paravento Elevado"
                      }
                      frame True {
                        # "Subir Parav."
                        n3014 = case shown="True" w3620 {
                          tunnel: [7 w3625] -> w3619
                          frame False {
                            w3624 = u16 4 items=["ZERO", "AH", "DEC", "TUBO", "CUP"] ("Controlador")
                            # "Aguardar subida Parav."
                            # "CLP Pronto"
                            n3015 = call "Monta Comando.vi"("Comando"="SUBIR", "Dispositivo"="PARAVENTO" ("Comando"), "Controlador"=w3624) -> ()  [unwired: 4 in, 3 out]
                          }
                          frame True {
                            # "CLP Busy"
                            n3016 = local read "TimeoutCUP 2"() -> (w3627:u32)
                            n3017 = call "TickTimeout.vi"("msInicial"=w3627, "msTimeout"=u32 5000) -> ("Timeout"=w3626:bool)  [unwired: 2 out]
                            n3018 = case shown="True" w3626 {
                              tunnel: [6 3] -> w3625
                              frame False {
                              }
                              frame True {
                              }
                            }
                          }
                        }
                      }
                    }
                  }
                  frame 7 {
                    w3632 = u16 7 items=["Alarme", "Atencao", "Erro", "Ocupado", "TBD", "LCB", "Trapeira", "Paravento", "DomoRap", "DomoCW", "DomoCCW", "TBD", "Em movimento", "TBD"] ("NomeStatus")
                    # "Também poderia ser testado o bit \"Em movimento\".\nNeste caso o código do \"IF\" deve ser permutado."
                    # "Aguarda Subida Paravento"
                    n3019 = call "Bit Status CUP.vi"("NomeStatus"=w3632) -> ("StatBit"=w3634:bool)
                    n3020 = Not(x=w3634) -> (.not. x?=w3631:bool)
                    n3021 = case shown="False" w3631 {
                      tunnel: [7 8] -> w3633
                      frame False {
                        # "Ainda movendo...\nAGUARDAR"
                      }
                      frame True {
                        # "Paravento elevado."
                      }
                    }
                  }
                  frame 8 {
                    # "CUP on target"
                    n3022 = local write "Dome on Target"(TRUE ("Dome on Target")) -> ()
                    n3023 = global write "Global_Telescopio.vi" "Parking"(FALSE) -> ()
                  }
                }
                n3024 = call "PROTECAO.vi"("Estado In"=w3526) -> ("Estado Out"=w3525:i32)  [unwired: 2 in]
                n3025 = Compound Arithmetic op=ADD(w3524, w3525, w3529, w3527) -> (w3535:i32)
                n3026 = Equal To 0?(x=w3535) -> (x = 0?=w3533:bool)
                n3027 = And(x=w3533, y=w3532) -> (x .and. y?=w3531:bool)
                n3028 = case shown="True" w3531 {
                  frame False {
                  }
                  frame True {
                    w3550 = FALSE
                    w3551 = u8 0 ("Disabled")
                    # "DESLIGA TODOS"
                    # "HABILITA TODOS"
                    n3029 = local write "BtUtilZenith"(w3550) -> ()
                    n3030 = local write "BtUtilPark"(w3550) -> ()
                    n3031 = local write "PROTEÇÃO"(w3550) -> ()
                    n3032 = local write "FLAT-FIELD"(w3550) -> ()
                    n3033 = local write "ECASS"(w3550) -> ()
                    n3034 = property on="BtUtilPark" class="Bool (strict)"("Disabled"=w3551) -> ()  [unwired: 2 in, 2 out]
                    n3035 = property on="ECASS" class="Bool (strict)"("Disabled"=w3551) -> ()  [unwired: 2 in, 2 out]
                    n3036 = property on="Setup, Pointing & Guiding" class="TabCtl (strict)"("Page Selector Visible"=TRUE) -> ()  [unwired: 2 in, 2 out]
                    n3037 = property on="BtUtilZenith" class="Bool (strict)"("Disabled"=w3551) -> ()  [unwired: 2 in, 2 out]
                    n3038 = property on="FLAT-FIELD" class="Bool (strict)"("Disabled"=w3551) -> ()  [unwired: 2 in, 2 out]
                    n3039 = property on="PROTEÇÃO" class="Bool (strict)"("Disabled"=w3551) -> ()  [unwired: 2 in, 2 out]
                  }
                }
                n3040 = local write "M_AH"(w3529) -> ()
                n3041 = local write "M_CUP"(w3525) -> ()
              }
              frame #4 {
                n3042 = case shown="True" "GO" {
                  frame False {
                  }
                  frame True {
                    w3934 = u16 3 items=["Alarme", "Atencao", "Erro", "Ocupado", "Protecao", "Embreagem", "Tracking", "Var. Track", "Rápido", "Ligeiro", "Médio", "Lento", "Em movimento", ""] ("NomeStatus")
                    w3935 = u16 3 items=["Alarme", "Atencao", "Erro", "Ocupado", "Protecao", "Embreagem", "Tracking", "Var. Track", "Rápido", "Ligeiro", "Médio", "Lento", "Em movimento", ""] ("NomeStatus")
                    n3043 = call "Bit Status AH.vi"("NomeStatus"=w3935) -> ("StatBit"=w3933:bool)
                    n3044 = call "Bit Status DEC.vi"("NomeStatus"=w3934) -> ("StatBit"=w3932:bool)
                    n3045 = Or(x=w3933, y=w3932) -> (x .or. y?=w3931:bool)
                    n3046 = case shown="False" w3931 {
                      frame False {
                        w3936 = FALSE ("RA on Target")
                        w3954 = u16 1 items=["ZERO", "AH", "DEC", "TUBO", "CUP"] ("Controlador")
                        w3959 = u16 2 items=["ZERO", "AH", "DEC", "TUBO", "CUP"] ("Controlador")
                        w3937 = FALSE ("GO")
                        n3047 = local write "RA on Target"(w3936) -> ()
                        n3048 = local write "DEC on Target"(w3936) -> ()
                        n3049 = global read "Global_Telescopio.vi" "Calagem AH"() -> (w3947:dbl)
                        n3050 = call "Comma_to_Point.vi"("Lat_A"="StrPointObjRA 2") -> ("Saída"=w3941:string)
                        n3051 = call "Comma_to_Point.vi"("Lat_A"="StrPointObjDEC 2") -> ("Saída"=w3938:string)
                        n3052 = global read "Global_Telescopio.vi" "Calagem DEC"() -> (w3946:dbl)
                        n3053 = call "hms_rad.vi"("True = hora"=TRUE, "Texto Graus"=w3941) -> ("radianos"=w3942:dbl)  [unwired: 3 in]
                        n3054 = call "hms_rad.vi"("True = hora"=FALSE, "Texto Graus"=w3938) -> ("radianos"=w3943:dbl)  [unwired: 3 in]
                        n3055 = Add(x=w3942, y=w3947) -> (x+y=w3945:dbl)
                        n3056 = Add(x=w3943, y=w3946) -> (x+y=w3944:dbl)
                        n3057 = local write "GO"(w3937) -> ()
                        n3058 = global write "Global_Telescopio.vi" "ObjCentrado"(w3937) -> ()
                        n3059 = call "rad_hms.vi"("TRUE=HORA\nFALSE=GRAU"=TRUE ("TRUE=HORA\nFALSE=GRAU"), "Radiano"=w3945) -> ("Hora/Graus Texto Decimal"=w3951:string)  [unwired: 3 in]
                        n3060 = call "rad_hms.vi"("TRUE=HORA\nFALSE=GRAU"=FALSE, "Radiano"=w3944) -> ("Hora/Graus Texto Decimal"=w3950:string)  [unwired: 3 in]
                        n3061 = call "Monta Comando.vi"("Set Point"=w3951, "Comando"="MOVER_ABS", "Dispositivo"="EIXO" ("Comando"), "Controlador"=w3954) -> ()  [unwired: 3 in, 3 out]
                        n3062 = call "Monta Comando.vi"("Set Point"=w3950, "Comando"="MOVER_ABS", "Dispositivo"="EIXO" ("Comando"), "Controlador"=w3959) -> ()  [unwired: 3 in, 3 out]
                      }
                      frame True {
                      }
                    }
                  }
                }
              }
            }
          }
        }
      }
      frame #3 {
        # "Desabiita Centragem\ndurante apontamento"
        # "PROCESSO TRACKING"
        # "Comando Via serial do Sist\nAquisição"
        # "CHAVES PAINEL"
        n3063 = disable-structure shown="Disabled" {
          frame Disabled {
            # "MUDANÇA 22MAR24:\nDados lidos apenas\ncom 0MQ."
            n3064 = case shown="True" "RESTART METEOR" {
              frame False {
              }
              frame True {
                n3065 = call "Teste_Read_Meteorologica.vi"() -> ("Erro"=w3978:bool)  [unwired: 2 in]
                n3066 = local write "Default Met"(w3978) -> ()
              }
            }
          }
          frame Enabled {
          }
        }
        n3067 = case shown="True" "BtShutterClose" {
          frame False {
          }
          frame True {
            w4005 = u16 3 items=["Alarme", "Atencao", "Erro", "Ocupado", "TBD", "LCB", "Trapeira", "Paravento", "DomoRap", "DomoCW", "DomoCCW", "TBD", "Em movimento", "TBD"] ("NomeStatus")
            n3068 = call "Bit Status CUP.vi"("NomeStatus"=w4005) -> ("StatBit"=w4006:bool)
            n3069 = case shown="False" w4006 {
              selector: w4006 -> [w4007 _]
              frame False {
                w4010 = u16 4 items=["ZERO", "AH", "DEC", "TUBO", "CUP"] ("Controlador")
                n3070 = local write "BtShutterClose"(w4007) -> ()
                n3071 = call "Monta Comando.vi"("Comando"="FECHAR", "Dispositivo"="TRAPEIRA" ("Comando"), "Controlador"=w4010) -> ()  [unwired: 4 in, 3 out]
              }
              frame True {
              }
            }
          }
        }
        n3072 = case shown="True" "Stop All" {
          frame False {
          }
          frame True {
